vi "HRTF-Enum Data Files.vi"(0 "State":T1, 7 "Azimuths":dbl[](array[numeric]), 11 "HRTFs":bool) -> (4 "filestems":string[](array[string]), 8 "file status":bool[][](array[boolean]))   [LabVIEW 2015]
uses:
  Typedefs/HRTF-State.ctl
  <vilib>/regexp/Match Regular Expression.xnode
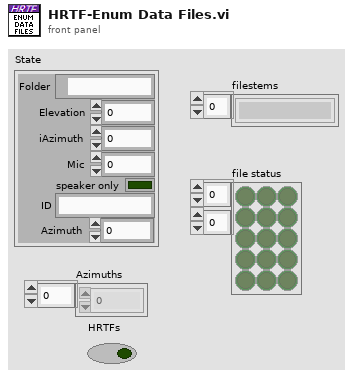
[diagram p1: front panel]
types:
  T1 = typedef "HRTF-State.ctl" = cluster{"Folder":path, "Elevation":dbl, "iAzimuth":i32, "Mic":i32, "speaker only":bool, "ID":string, "Azimuth":dbl}
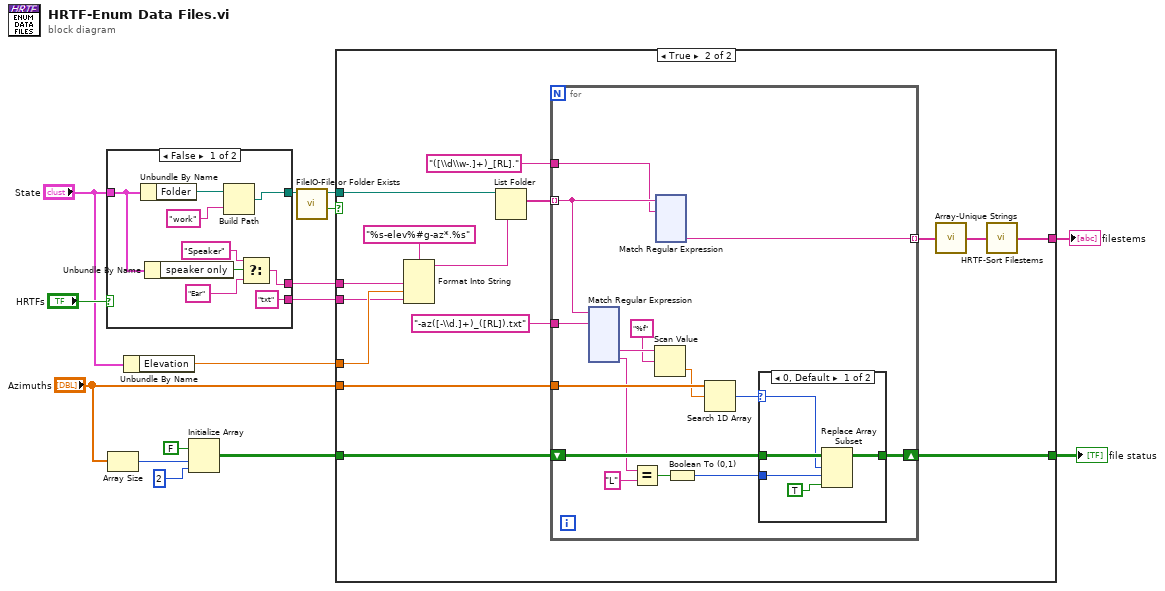
[diagram p0: block diagram]
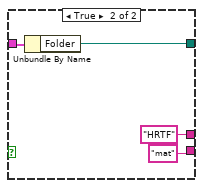
[diagram p2: hidden frame]
diagram:
  n1 = case shown="False" "HRTFs" {
    tunnel: [w21 "HRTF"] -> w15
    tunnel: ["txt" "mat"] -> w4
    tunnel: "State" -> [w19 w26]
    tunnel: [w17 w25] -> w1
    frame False {
      n2 = Unbundle By Name(w19) -> ("Folder"=w18:path)
      n3 = Unbundle By Name(w19) -> ("speaker only"=w24:bool)
      n4 = Build Path(base path=w18, name or relative path="work") -> (appended path=w17:path)
      n5 = Select(t="Speaker", s=w24, f="Ear") -> (s? t:f=w21:string)
    }
    frame True {
      n6 = Unbundle By Name(w26) -> ("Folder"=w25:path)
    }
  }
  n7 = Array Size(array="Azimuths") -> (size(s)=w7:i32)
  n8 = Unbundle By Name("State") -> ("Elevation"=w5:dbl)
  n9 = Initialize Array(FALSE, w7, 2 ("dimension size")) -> (w13:bool[][])
  n10 = call "FileIO-File or Folder Exists.vi"("path"=w1) -> ("Exists?"=w8:bool, "dup path"=w9:path)  [unwired: 7 in, 2 out]
  n11 = case shown="True" w8 {
    tunnel: w15 -> [_ w43]
    tunnel: w5 -> [_ w42]
    tunnel: w9 -> [_ w41]
    tunnel: w13 -> [w29 w38]
    tunnel: "Azimuths" -> [_ w37]
    tunnel: [w29 w35] -> w11
    tunnel: [_ w30] -> w10
    tunnel: w4 -> [_ w32]
    frame False {
    }
    frame True {
      n12 = Format Into String(format string="%s-elev%#g-az*.%s", w43, w42, w32) -> (resulting string=w40:string)  [unwired: 2 in, 1 out]
      n13 = List Folder(path=w41, pattern=w40) -> (filenames=w39:string[])  [unwired: 2 in, 3 out]
      n14 = for {
        tunnel: w39 -> [w50] mode=indexing
        shift-right: [w55] -> w35
        shift-left: w38 -> [w56]
        tunnel: w37 -> [w58]
        tunnel: "-az([-\\d.]+)_([RL]).txt" ("regular expression") -> [w59]
        tunnel: "([\\d\\w-.]+)_[RL]." -> [w49]
        tunnel: [w48] -> w33 mode=indexing
        n15 = xnode "Match Regular Expression"("input string"=w50, "regular expression"=w59) -> ("submatch 1"=w47:string, "submatch 2"=w46:string)  [unwired: 4 in, 5 out]
        n16 = Equal?(x=w46, y="L") -> (x = y?=w52:bool)
        n17 = Scan Value(string=w47, format string="%f") -> (value=w57:dbl)  [unwired: 1 in, 1 out]
        n18 = xnode "Match Regular Expression"("input string"=w50, "regular expression"=w49) -> ("submatch 1"=w48:string)  [unwired: 4 in, 5 out]
        n19 = Boolean To (0,1)(Boolean=w52) -> (0, 1=w51:i16)
        n20 = Search 1D Array(1D array=w58, element=w57) -> (index of element=w54:i32)  [unwired: 1 in]
        n21 = case shown="0, Default" w54 {
          selector: w54 -> [w177 _]
          tunnel: w56 -> [w180 w181]
          tunnel: [w179 w181] -> w55
          tunnel: w51 -> [w176 _]
          frame 0, Default {
            n22 = Replace Array Subset(array=w180, new element=TRUE ("new element/subarray"), index (row)=w177, index (col)=w176) -> (w179:bool[][])
          }
          frame -1 {
          }
        }
      }
      n23 = call "Array-Unique Strings.vi"("Strings"=w33) -> ("Unique strings"=w31:string[])  [unwired: 4 in]
      n24 = call "HRTF-Sort Filestems.vi"("Filestems"=w31) -> ("Sorted filestems"=w30:string[])  [unwired: 14 in]
    }
  }
  "file status" <- w11
  "filestems" <- w10
